vi "Post_Pro_Results_Hierarchy.vi"() -> ()   [LabVIEW 2022 SP3]
uses:
  Anemometry Sub Vis/Globals/Meas_global.vi
  Anemometry Sub Vis/Globals/Plug_in_data_global.vi
panel:
  out "Seconds Taken":dbl format="%#.0f"
  in  "Choose Plug Ins":bool
  in  "Per Block Plug Ins Extra":string[](array[string])
  in  "Template":path
  out "Current File Number":i32
  out "Number of Files to Process":i32
  out "Currently Processing":path
  out "Files to Post Process":path[](array[path])
  in  "Save results to":T1(ring)=enum."Original Results Filenames"
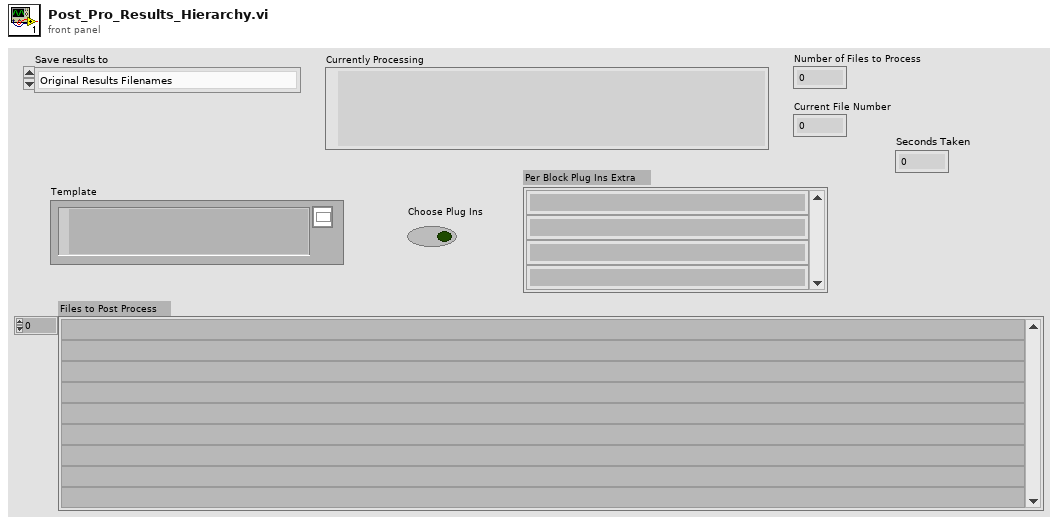
[diagram p1: front panel]
types:
  T1 = enum16{"A single file", "Original Results Filenames", "Current Results Filenames"}
  T2 = enum16{"Zero or one", "One", "Zero or more", "One or more"}
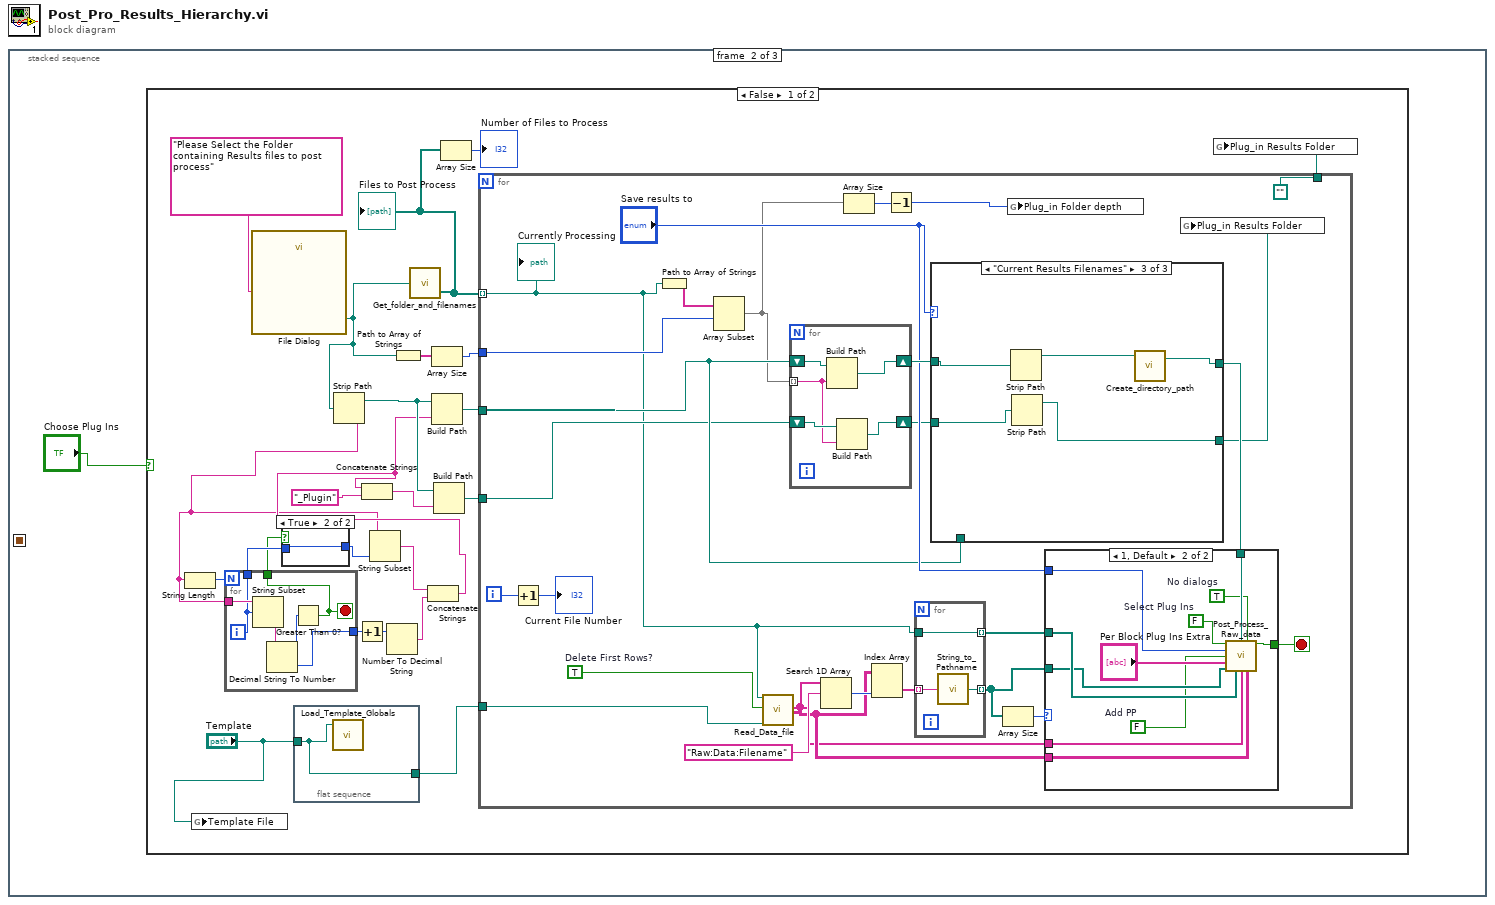
[diagram p0: block diagram]
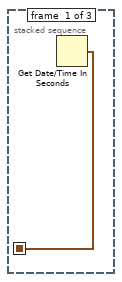
[diagram p2: hidden frame]
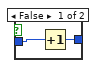
[diagram p3: hidden frame]
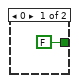
[diagram p4: hidden frame]
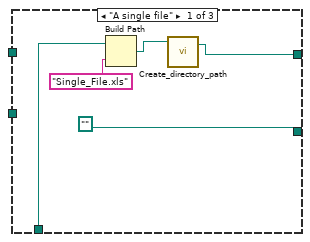
[diagram p5: hidden frame]
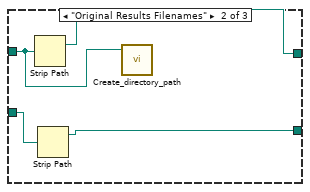
[diagram p6: hidden frame]
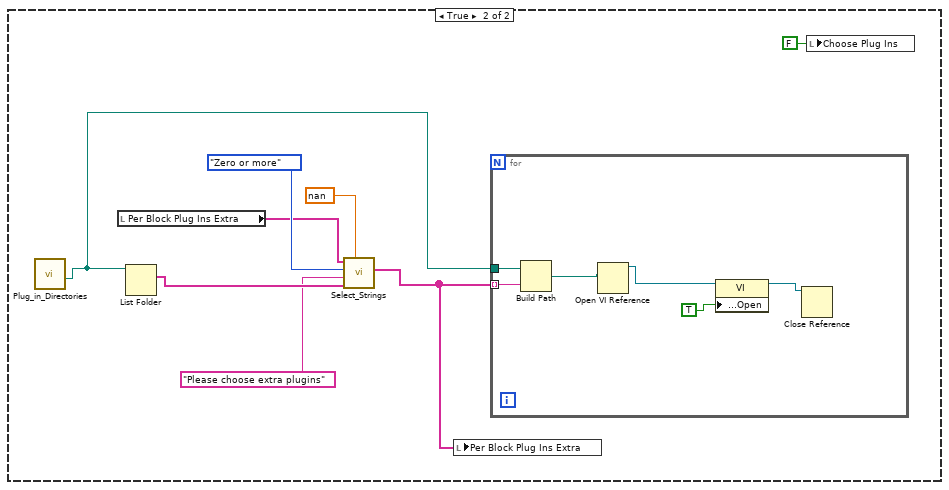
[diagram p7: hidden frame]
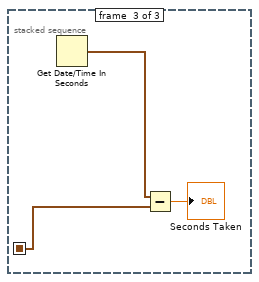
[diagram p8: hidden frame]
diagram:
  n1 = stacked-sequence {
    seq-local: [w1 _ _] -> [_ _ w113]
    frame #0 {
      n2 = Get Date/Time In Seconds() -> (seconds since 1Jan1904=w1:timestamp)
    }
    frame #1 {
      n3 = case shown="False" "Choose Plug Ins" {
        frame False {
          n4 = global write "Meas_global.vi" "Template File"("Template") -> ()
          n5 = call "File Dialog"("prompt"="Please Select the Folder containing Results files to post process") -> ("selected path"=w23:path)  [unwired: 11 in, 3 out]
          n6 = flat-sequence {
            tunnel: "Template" -> [w36]
            tunnel: [w36] -> w14
            frame #0 {
              n7 = call "Load_Template_Globals.vi"("Template-read"=w36) -> ()  [unwired: 2 in, 1 out]
            }
          }
          n8 = Strip Path(path=w23) -> (stripped path=w19:path, name=w4:string)
          n9 = String Length(string=w4) -> (length=w13:i32)
          n10 = for {
            N: w13 -> [_]
            tunnel: w4 -> [w35]
            tunnel: [w32] -> w12
            tunnel: [w31] -> w7
            tunnel: [w30] -> w6
            i -> [w31]
            stop <- w30 stop-if-true
            n11 = String Subset(string=w35, offset (0)=w31) -> (substring=w34:string)  [unwired: 1 in]
            n12 = Decimal String To Number(string=w34) -> (offset past number=w33:i32, number=w32:i32)  [unwired: 2 in]
            n13 = Greater Than 0?(x=w33) -> (x > 0?=w30:bool)
          }
          n14 = case shown="True" w6 {
            tunnel: [w28 w29] -> w8
            tunnel: w7 -> [w27 w29]
            frame False {
              n15 = Increment(x=w27) -> (x+1=w28:i32)
            }
            frame True {
            }
          }
          n16 = Increment(x=w12) -> (x+1=w11:i32)
          n17 = String Subset(string=w4, length (rest)=w8) -> (substring=w10:string)  [unwired: 1 in]
          n18 = Number To Decimal String(number=w11) -> (decimal integer string=w9:string)  [unwired: 1 in]
          n19 = Path to Array of Strings(0:w23) -> (2:w25:string[])  [unwired: 1 out]
          n20 = call "Get_folder_and_filenames.vi"("file path (dialog if empty)"=w23) -> ("Files"=w21:path[])  [unwired: 1 out]
          "Files to Post Process" <- w21
          n21 = Concatenate Strings(w10, w9) -> (w5:string)
          n22 = Concatenate Strings(w5, "_Plugin" ("string")) -> (w17:string)
          n23 = Array Size(array=w25) -> (size(s)=w24:i32)
          n24 = Build Path(base path=w19, name or relative path=w5) -> (appended path=w22:path)
          n25 = Build Path(base path=w19, name or relative path=w17) -> (appended path=w16:path)
          n26 = Array Size(array=w21) -> (size(s)=→"Number of Files to Process":i32)
          n27 = for {
            tunnel: w21 -> [w48] mode=indexing
            tunnel: w24 -> [w62]
            tunnel: w22 -> [w59]
            tunnel: w16 -> [w55]
            tunnel: w14 -> [w42]
            tunnel: [path ""] -> w15
            i -> [w57]
            stop <- w43 stop-if-true
            w49 = TRUE  # Delete First Rows?
            n28 = Increment(x=w57) -> (x+1=→"Current File Number":i32)
            n29 = Path to Array of Strings(0:w48) -> (2:w63:string[])  [unwired: 1 out]
            n30 = Array Subset(array=w63, index=w62) -> (w41:string[])  [unwired: 1 in]
            n31 = call "Read_Data_file.vi"("Results file"=w48, "Delete First Rows?"=w49, "Template File"=w42) -> ("Ch names Out"=w44:string[], "Channel Values Out"=w45:string[][])  [unwired: 4 in, 11 out]
            n32 = for {
              tunnel: w41 -> [w93] mode=indexing
              shift-right: [w96] -> w61
              shift-left: w59 -> [w97]
              shift-right: [w95] -> w53
              shift-left: w55 -> [w94]
              n33 = Build Path(base path=w97, name or relative path=w93) -> (appended path=w96:path)
              n34 = Build Path(base path=w94, name or relative path=w93) -> (appended path=w95:path)
            }
            n35 = Search 1D Array(1D array=w44, element="Raw:Data:Filename") -> (index of element=w51:i32)  [unwired: 1 in]
            n36 = Array Size(array=w41) -> (size(s)=w40:i32)
            n37 = Index Array(array=w45, index (col)=w51) -> (element=w52:string[])  [unwired: 1 in]
            n38 = Decrement(x=w40) -> (x-1=w39:i32)
            n39 = for {
              tunnel: w52 -> [w78] mode=indexing
              tunnel: [w77] -> w37 mode=indexing
              tunnel: [w76] -> w47 mode=indexing
              tunnel: w48 -> [w76]
              n40 = call "String_to_Pathname.vi"("Input String"=w78) -> ("path"=w77:path)
            }
            n41 = case shown="\"Current Results Filenames\"" "Save results to" {
              tunnel: w61 -> [_ w85 w91]
              tunnel: [w80 w86 w92] -> w58
              tunnel: w59 -> [w83 _ _]
              tunnel: [path "" w84 w88] -> w54
              tunnel: w53 -> [_ w87 w89]
              frame "A single file" {
                n42 = Build Path(base path=w83, name or relative path="Single_File.xls") -> (appended path=w81:path)
                n43 = call "Create_directory_path.vi"("Path name"=w81) -> ("Path name Out"=w80:path)  [unwired: 2 in, 1 out]
              }
              frame "Original Results Filenames" {
                n44 = Strip Path(path=w85) -> (stripped path=w86:path)  [unwired: 1 out]
                n45 = Strip Path(path=w87) -> (stripped path=w84:path)  [unwired: 1 out]
                n46 = call "Create_directory_path.vi"("Path name"=w85) -> ()  [unwired: 2 in, 2 out]
              }
              frame "Current Results Filenames" {
                n47 = Strip Path(path=w91) -> (stripped path=w90:path)  [unwired: 1 out]
                n48 = Strip Path(path=w89) -> (stripped path=w88:path)  [unwired: 1 out]
                n49 = call "Create_directory_path.vi"("Path name"=w90) -> ("Path name Out"=w92:path)  [unwired: 2 in, 1 out]
              }
            }
            n50 = Array Size(array=w37) -> (size(s)=w38:i32)
            n51 = global write "Plug_in_data_global.vi" "Plug_in Folder depth"(w39) -> ()
            n52 = case shown="1, Default" w38 {
              tunnel: "Save results to" -> [_ w75]
              tunnel: w58 -> [_ w74]
              tunnel: w47 -> [_ w73]
              tunnel: w37 -> [_ w72]
              tunnel: w45 -> [_ w71]
              tunnel: w44 -> [_ w70]
              tunnel: [FALSE ("Stopped") w66] -> w43
              frame 0 {
              }
              frame 1, Default {
                w65 = FALSE  # Add PP
                w68 = TRUE  # No dialogs
                w69 = FALSE  # Select Plug Ins
                n53 = call "Post_Process_Raw_data.vi"("Select Plug Ins"=w69, "Post processed Results folder"=w74, "No dialogs"=w68, "Save results to"=w75, "Add PP"=w65, "Per Block Plug Ins Extra"="Per Block Plug Ins Extra", "Selected files"=w72, "Current Results filenames"=w73, "Results Plotter Channel names"=w70, "Results Plotter Data"=w71) -> ("Stopped"=w66:bool)  [unwired: 4 in, 1 out]
              }
            }
            n54 = global write "Plug_in_data_global.vi" "Plug_in Results Folder"(w54) -> ()
            "Currently Processing" <- w48
          }
          n55 = global write "Plug_in_data_global.vi" "Plug_in Results Folder"(w15) -> ()
        }
        frame True {
          n56 = call "Plug_in_Directories.vi"() -> ("Per Block"=w100:path)  [unwired: 2 in, 4 out]
          n57 = local read "Per Block Plug Ins Extra"() -> (w103:string[])
          n58 = List Folder(path=w100) -> (filenames=w104:string[])  [unwired: 3 in, 3 out]
          n59 = call "Select_Strings.vi"("Timeout (s)"=nan, "Available Ch names"=w104, "Message"="Please choose extra plugins", "Selector mode"=T2."Zero or more", "Desired Ch names (in)"=w103) -> ("Selected Channel Names"=w99:string[])  [unwired: 1 in, 2 out]
          n60 = local write "Per Block Plug Ins Extra"(w99) -> ()
          n61 = for {
            tunnel: w100 -> [w111]
            tunnel: w99 -> [w106] mode=indexing
            n62 = Build Path(base path=w111, name or relative path=w106) -> (appended path=w110:path)
            n63 = Open VI Reference(vi path=w110) -> (vi reference=w108:refnum<vi>)  [unwired: 5 in, 1 out]
            n64 = property class="VI"(reference=w108, "Front Panel Window:Open"=TRUE) -> (reference out=w107:refnum<vi>)  [unwired: 1 in, 1 out]
            n65 = Close Reference(reference=w107) -> ()  [unwired: 1 in, 1 out]
          }
          n66 = local write "Choose Plug Ins"(FALSE ("Choose Plug Ins")) -> ()
        }
      }
    }
    frame #2 {
      n67 = Get Date/Time In Seconds() -> (seconds since 1Jan1904=w114:timestamp)
      n68 = Subtract(x=w114, y=w113) -> (x-y=→"Seconds Taken":dbl)
    }
  }
